vi "specialUrlEncode.vi"(11 "str":string) -> (3 "UrlEncode":string)   [LabVIEW 2016, in "数据传输系统-03.lvlib" / "update.lvlib"]
uses:
  update.lvlib
  System.Web
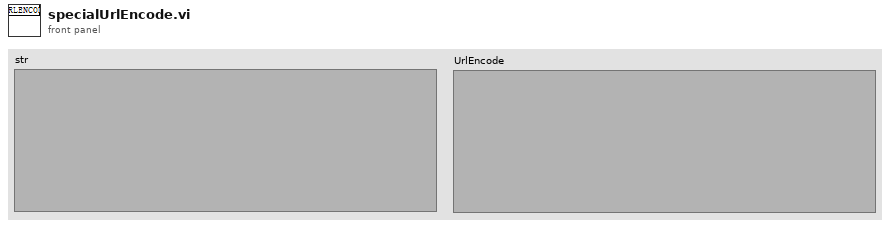
[diagram p1: front panel]
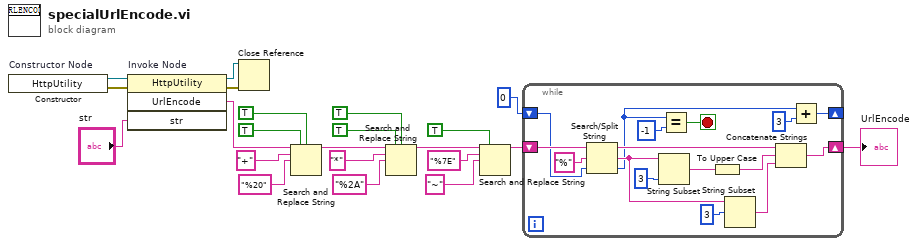
[diagram p0: block diagram]
diagram:
  n1 = constructor on="Constructor Node" class="HttpUtility"() -> (reference out=w22:refnum<k24>, error out=w21:errorcluster)  [unwired: 3 in, 1 out]
  n2 = invoke on="Invoke Node" class="HttpUtility" method="UrlEncode"(reference=w22, error in=w21, "str"="str") -> (reference out=w19:refnum<k24>, error out=w20:errorcluster, "UrlEncode"=w4:string)  [unwired: 1 in, 1 out]
  n3 = Close Reference(reference=w19, error in (no error)=w20) -> ()  [unwired: 1 out]
  n4 = Search and Replace String(replace all?=TRUE ("替换全部？(F)"), case sensitive?=TRUE ("忽略大小写？(F)"), input string=w4, search string="+" ("搜索字符串"), replace string="%20" ("替换字符串(\"\")")) -> (result string=w3:string)  [unwired: 3 in, 3 out]
  n5 = Search and Replace String(replace all?=TRUE ("替换全部？(F)"), case sensitive?=TRUE ("忽略大小写？(F)"), input string=w3, search string="*" ("搜索字符串"), replace string="%2A" ("替换字符串(\"\")")) -> (result string=w13:string)  [unwired: 3 in, 3 out]
  n6 = Search and Replace String(replace all?=TRUE ("替换全部？(F)"), input string=w13, search string="%7E" ("搜索字符串"), replace string="~" ("替换字符串(\"\")")) -> (result string=w7:string)  [unwired: 4 in, 3 out]
  n7 = while {
    shift-right: [w28] -> w8
    shift-left: w7 -> [w38]
    shift-right: [w34] -> _
    shift-left: 0 -> [w36]
    stop <- w25 stop-if-true
    n8 = Search/Split String(string=w38, search string/char (-)="%" ("搜索字符串/字符(-)"), offset (0)=w36) -> (substring before match=w30:string, match + rest of string=w32:string, offset of match=w27:i32)
    n9 = String Subset(string=w32, length (rest)=3 ("长度（剩余）")) -> (substring=w24:string)  [unwired: 1 in]
    n10 = Equal?(x=w27, y=-1) -> (x = y?=w25:bool)
    n11 = To Upper Case(1:w24) -> (0:w23:string)
    n12 = String Subset(string=w32, offset (0)=3 ("偏移量(0)")) -> (substring=w29:string)  [unwired: 1 in]
    n13 = Concatenate Strings(w30, w23, w29) -> (w28:string)
    n14 = Add(x=w27, y=3) -> (x+y=w34:i32)
  }
  "UrlEncode" <- w8
